vi "rad_Configure Individual Bitfile Settings Dialog.vi"(8 "error in (no error)":errorcluster, 10 "Default RIO Resource":string, 11 "FPGA Properties":T1) -> (0 "error out":errorcluster, 2 "Canceled":bool, 3 "FPGA Properties Out":T1)   [LabVIEW 2013]
uses:
  TypeDefs/rad_FPGA Flash Properties.ctl
  Util/FP Control/FP Control Functions.ctl
panel:
  in  "Cancel":bool
  in  "OK":bool
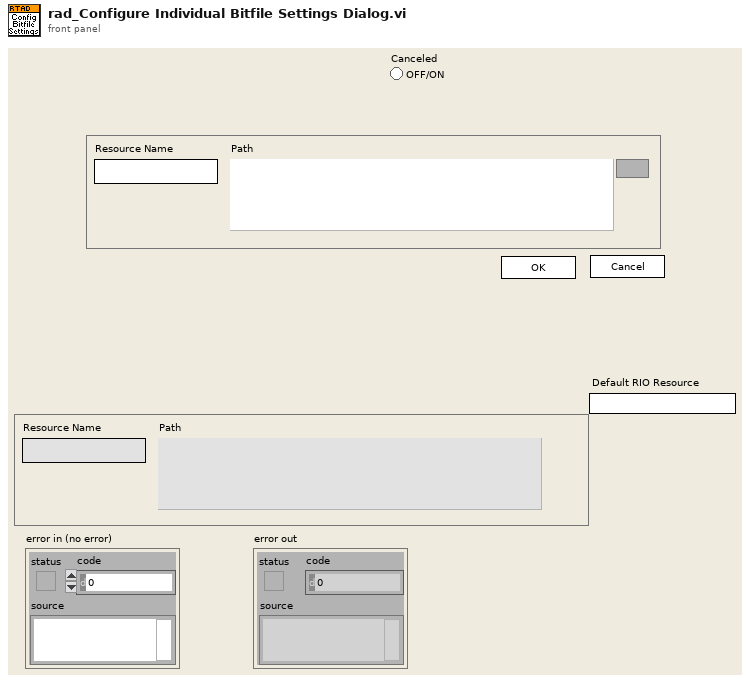
[diagram p1: front panel]
types:
  T1 = typedef "rad_FPGA Flash Properties.ctl" = cluster{"Resource Name":string, "Path":path}
  T2 = typedef "FP Control Functions.ctl" = enum16{"Open", "Close", "Bring To Front", "Center"}
  T3 = enum8{"Enabled", "Disabled", "Disabled and Grayed Out"}
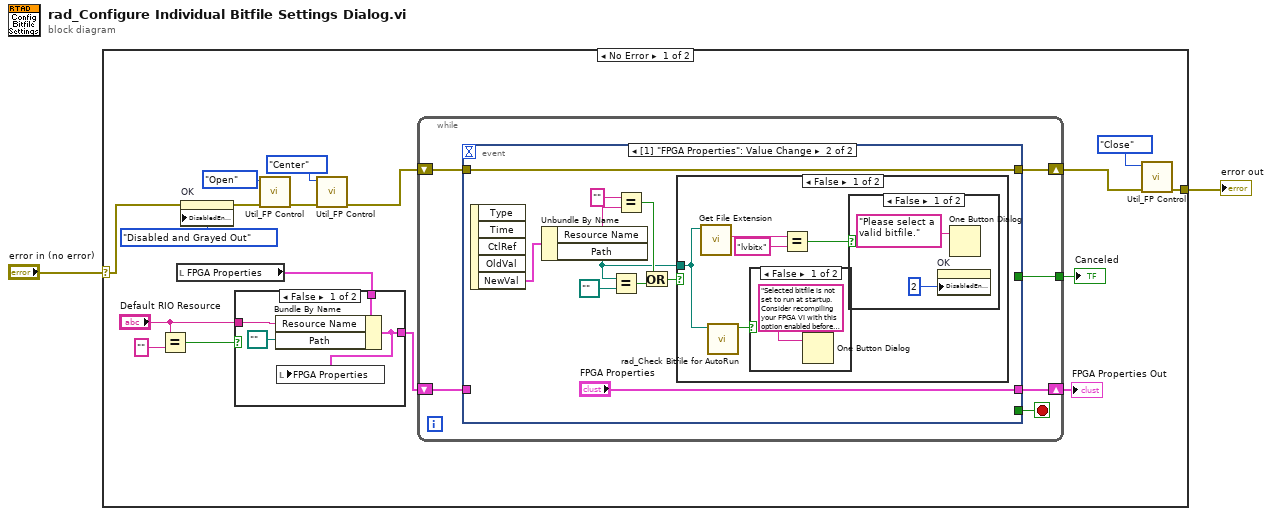
[diagram p0: block diagram]
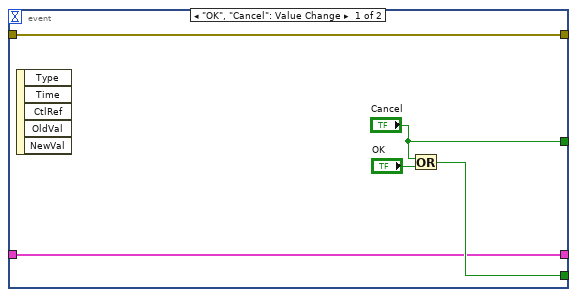
[diagram p2: hidden frame]
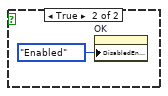
[diagram p4: hidden frame]
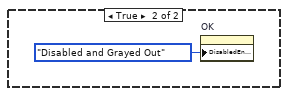
[diagram p5: hidden frame]
diagram:
  n1 = case shown="No Error" "error in (no error)" {
    selector: "error in (no error)" -> [w3 w56]
    tunnel: [w7 w56] -> w2
    frame No Error {
      n2 = Equal?(x="Default RIO Resource", y="") -> (x = y?=w13:bool)
      n3 = local read "FPGA Properties"() -> (w15:T1)
      n4 = property on="OK" class="Bool"(error in=w3, "DisabledEnum"=T3."Disabled and Grayed Out" ("Disabled")) -> (error out=w11:errorcluster)  [unwired: 1 in, 1 out]
      n5 = case shown="False" w13 {
        tunnel: [w53 w55] -> w18
        tunnel: w15 -> [w52 w55]
        tunnel: "Default RIO Resource" -> [w51 _]
        frame False {
          n6 = Bundle By Name(cluster=w52, "Resource Name"=w51, "Path"=path "") -> (w53:T1)
          n7 = local write "FPGA Properties"(w53) -> ()
        }
        frame True {
        }
      }
      n8 = call "Util_FP Control.vi"("error in (no error)"=w11, "Function"=FP_Control_Functions."Open") -> ("error out"=w10:errorcluster)  [unwired: 9 out]
      n9 = call "Util_FP Control.vi"("error in (no error)"=w10, "Function"=FP_Control_Functions."Center") -> ("error out"=w16:errorcluster)  [unwired: 9 out]
      n10 = while {
        tunnel: [w22] -> w5
        shift-right: [w24] -> w6
        shift-left: w18 -> [w25]
        shift-right: [w20] -> w8
        shift-left: w16 -> [w21]
        stop <- w23 stop-if-true
        n11 = event shown="[1] \"FPGA Properties\": Value Change" {
          selector: _ -> [_ _]
          dyn-events: _ -> [_ _]
          timeout: _ -> [_ _]
          tunnel: w25 -> [w27 _]
          tunnel: [w27 "FPGA Properties"] -> w24
          tunnel: [w29 _] -> w23
          tunnel: ["Cancel" _] -> w22
          tunnel: w21 -> [w26 w31]
          tunnel: [w26 w31] -> w20
          event "OK", "Cancel": Value Change {
            n12 = event-data() -> ()  [unwired: 1 in, 5 out]
            n13 = Or(x="Cancel", y="OK") -> (x .or. y?=w29:bool)
          }
          event Value Change {
            n14 = event-data() -> ("NewVal"=w39:T1)  [unwired: 1 in, 4 out]
            n15 = Unbundle By Name(w39) -> ("Resource Name"=w38:string, "Path"=w32:path)
            n16 = Equal?(x=w32, y=path "") -> (x = y?=w36:bool)
            n17 = Equal?(x="", y=w38) -> (x = y?=w35:bool)
            n18 = Or(x=w35, y=w36) -> (x .or. y?=w34:bool)
            n19 = case shown="False" w34 {
              tunnel: w32 -> [w42 _]
              frame False {
                n20 = call <vilib>:"Get File Extension.vi"("file"=w42) -> ("lowercase file extension"=w45:string)  [unwired: 7 in, 3 out]
                n21 = call "rad_Check Bitfile for AutoRun.vi"("path to XML document"=w42) -> ("AutoRun?"=w41:bool)  [unwired: 8 in, 2 out]
                n22 = case shown="False" w41 {
                  frame False {
                    n23 = One Button Dialog(message="Selected bitfile is not set to run at startup.  Consider recompiling your FPGA VI with this option enabled before using this feature.") -> ()  [unwired: 1 in, 1 out]
                  }
                  frame True {
                  }
                }
                n24 = Equal?(x=w45, y="lvbitx") -> (x = y?=w43:bool)
                n25 = case shown="False" w43 {
                  frame False {
                    n26 = property on="OK" class="Bool"("DisabledEnum"=2) -> ()  [unwired: 2 in, 2 out]
                    n27 = One Button Dialog(message="Please select a valid bitfile.") -> ()  [unwired: 1 in, 1 out]
                  }
                  frame True {
                    n28 = property on="OK" class="Bool"("DisabledEnum"=T3."Enabled" ("Disabled")) -> ()  [unwired: 2 in, 2 out]
                  }
                }
              }
              frame True {
                n29 = property on="OK" class="Bool"("DisabledEnum"=T3."Disabled and Grayed Out" ("Disabled")) -> ()  [unwired: 2 in, 2 out]
              }
            }
          }
        }
      }
      "FPGA Properties Out" <- w6
      "Canceled" <- w5
      n30 = call "Util_FP Control.vi"("error in (no error)"=w8, "Function"=FP_Control_Functions."Close") -> ("error out"=w7:errorcluster)  [unwired: 9 out]
    }
    frame Error {
    }
  }
  "error out" <- w2
